vi "Set NodeID Ign.vi"(8 "error in (no error)":errorcluster, 10 "Control ref":refnum<vi>, 11 "folder name":string="NonUDT") -> (0 "error out":errorcluster, 3 "NodeIDs":string[](array[string]))   [LabVIEW 2019, in "Ignition.lvlib"]
uses:
  Ignition.lvlib
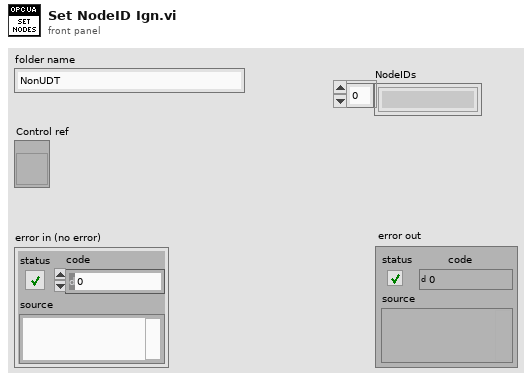
[diagram p1: front panel]
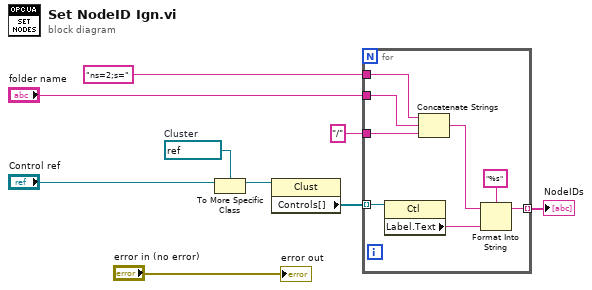
[diagram p0: block diagram]
diagram:
  w5 = refnum<vi> refnum  # Cluster
  n1 = To More Specific Class(target class=w5, reference="Control ref") -> (specific class reference=w4:refnum<vi>)  [unwired: 1 in, 1 out]
  n2 = property class="Clust"(reference=w4) -> ("Controls[]"=w6:refnum<vi>[])  [unwired: 1 in, 2 out]
  n3 = for {
    tunnel: w6 -> [w17] mode=indexing
    tunnel: "folder name" -> [w13]
    tunnel: [w14] -> w1 mode=indexing
    tunnel: "ns=2;s=" ("format string") -> [w12]
    tunnel: "/" ("Deliminated Char") -> [w10]
    n4 = property class="Ctl"(reference=w17) -> ("Label.Text"=w16:string)  [unwired: 1 in, 2 out]
    n5 = Concatenate Strings(w12, w13, w10) -> (w11:string)
    n6 = Format Into String(format string="%s", initial string=w11, w16) -> (resulting string=w14:string)  [unwired: 1 in, 1 out]
  }
  "NodeIDs" <- w1
  "error out" <- "error in (no error)"
